vi "Operator.vi"(8 "error in (no error)":errorcluster, 11 "Logical And in":refnum<class "Logical And.lvclass">) -> (0 "error out":errorcluster, 2 "Operator":string, 3 "Logical And out":refnum<class "Logical And.lvclass">)   [LabVIEW 2017, in "Transparent Assertions.lvlib" / "Constraints.lvlib" / "Logical And.lvclass"]
uses:
  Logical And.lvclass
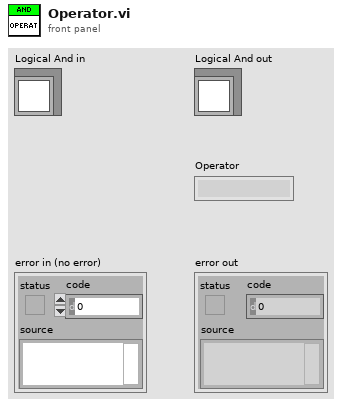
[diagram p1: front panel]
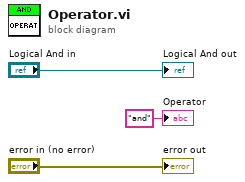
[diagram p0: block diagram]
diagram:
  "error out" <- "error in (no error)"
  "Logical And out" <- "Logical And in"
  "Operator" <- "and" ("Operator")
